vi "手动启动选择对话框.vi"() -> (2 "确定":bool, 3 "输出簇":cluster{"参数启用":T1})   [LabVIEW 2016, in "PLC.lvlib"]
uses:
  PLC.lvlib
  <vilib>/Utility/miscctls.llb/LVPointTypeDef.ctl
panel:
  in  "自动运行启动参数":T1
  in  "取消":bool
  in  "确定":bool
  # "请选择启动参数"
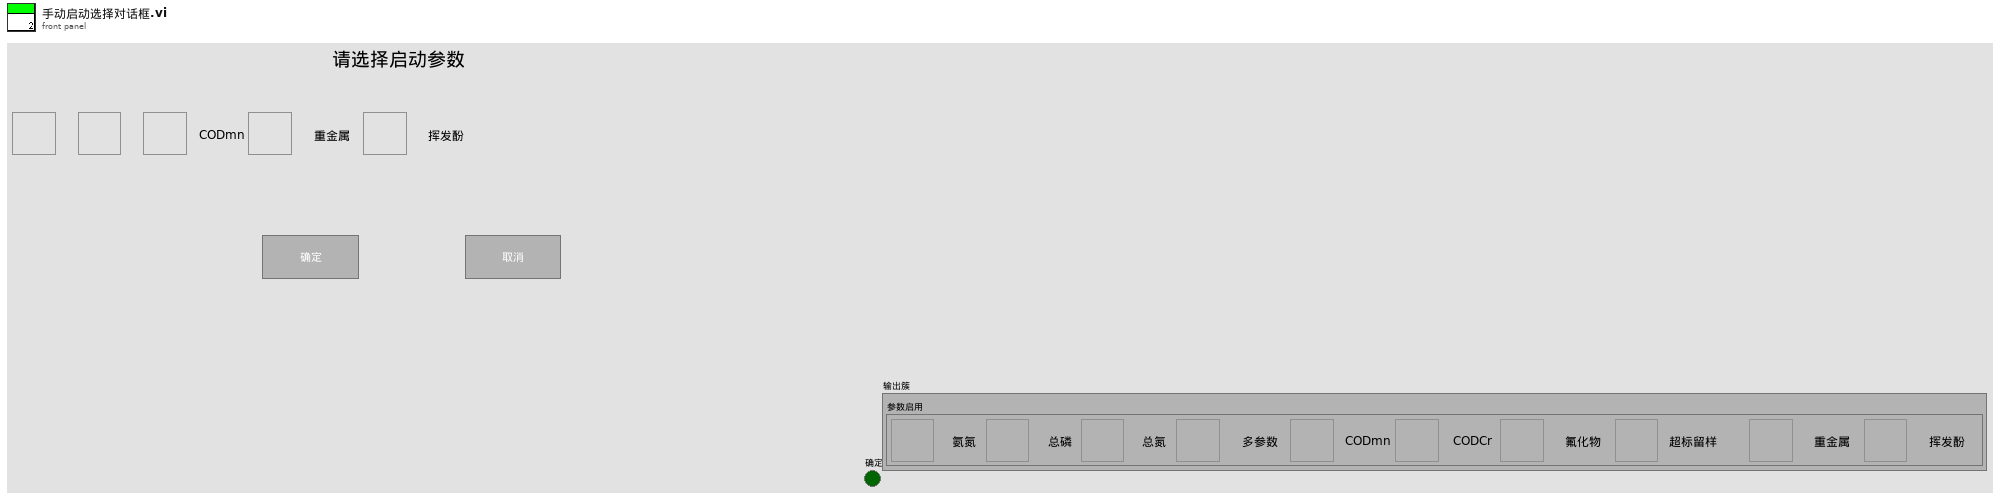
[diagram p1: front panel]
types:
  T1 = typedef "启动参数.ctl" = cluster{"氨氮":bool, "总磷":bool, "总氮":bool, "多参数":bool, "CODmn":bool, "CODCr":bool, "氟化物":bool, "超标留样启用":bool, "重金属":bool, "挥发酚":bool}
  T2 = typedef "LVPointTypeDef.ctl" = cluster{"Horizontal":i16, "Vertical":i16}
  T3 = typedef "模块配置类型.ctl" = enum16{"单模块", "总磷总氮二合一模块", "氨氮总磷二合一模块"}
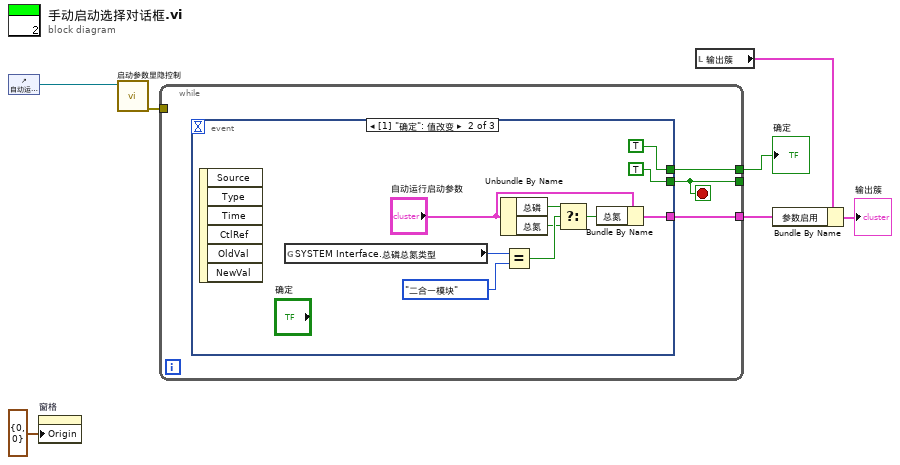
[diagram p0: block diagram]
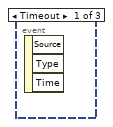
[diagram p2: hidden frame]
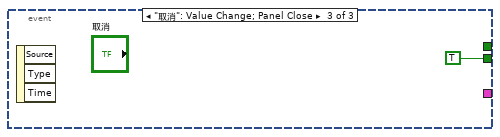
[diagram p3: hidden frame]
diagram:
  n1 = control-ref of="自动运行启动参数"() -> (w2:refnum<vi>)
  n2 = property on="窗格" class="Pane"("Origin"=T2 {"Horizontal"=0, "Vertical"=0} ("原点")) -> ()  [unwired: 2 in, 2 out]
  n3 = call "启动参数显隐控制.vi"("控件"=w2) -> ("error out"=w1:errorcluster)  [unwired: 10 in]
  n4 = while {
    tunnel: [w10] -> w6
    tunnel: [w9] -> _
    tunnel: [w8] -> w7
    tunnel: w1 -> [_]
    stop <- w9 stop-if-true
    n5 = event shown="[1] \"确定\": 值改变" {
      selector: _ -> [_ _ _]
      dyn-events: _ -> [_ _ _]
      timeout: _ -> [_ _ _]
      tunnel: [_ TRUE TRUE] -> w9
      tunnel: [_ w17 _] -> w10
      tunnel: [_ TRUE _] -> w8
      event Timeout {
        n6 = event-data() -> ()  [unwired: 1 in, 3 out]
      }
      event "确定": Value Change {
        n7 = event-data() -> ()  [unwired: 1 in, 6 out]
        n8 = global read "系统设置全局变量.vi" "SYSTEM Interface.总磷总氮类型"() -> (w16:T3)
        n9 = Unbundle By Name("自动运行启动参数") -> ("总磷"=w13:bool, "总氮"=w12:bool)
        n10 = Equal?(x=w16, y=enum16{"单模块", "二合一模块"}."二合一模块") -> (x = y?=w14:bool)
        n11 = Select(t=w13, s=w14, f=w12) -> (s? t:f=w11:bool)
        n12 = Bundle By Name(cluster="自动运行启动参数", "总氮"=w11) -> (w17:T1)
      }
      event "取消": Value Change; Panel Close {
        n13 = event-data() -> ()  [unwired: 1 in, 3 out]
      }
    }
  }
  "确定" <- w7
  n14 = local read "输出簇"() -> (w5:cluster{"参数启用":T1})
  n15 = Bundle By Name(cluster=w5, "参数启用"=w6) -> (→"输出簇":cluster{"参数启用":T1})
